vi "Configure AI.vi"(5 "Purpose (\"AI\")":string="AI", 7 "ADC #":T1=-1, 8 "error in (no error)":errorcluster, 11 "Session in":refnum<class "Session.lvclass">) -> (0 "error out":errorcluster, 3 "Session out":refnum<class "Session.lvclass">)   [LabVIEW 2024, in "CTI.lvlib" / "Session.lvclass"]
doc: "Configures a pin on the device to be used as an analog input. Unlike most other resource configuration VIs, the analog input is specified by its ADC number which can be found on the pinout for your device. Analog inputs are used to read a voltage value. When using these base AI features of the driver the raw integer reading will be returned which requires scaling to a proper voltage or engineering units and will depend on the wiring and configuration of the AI.\n\nThe Purpose input can be used to help with error reporting and provide a more specific intended use of the ADC that will be shown in future error messages resulting from I/O pin conflicts."
uses:
  Session.lvclass
  ADC Number.ctl
  Session.lvclass/Session.ctl
  2e1a53d0-5087-401c-a7a1-0aa9efa88061.vi
  Is Full Errors.vi
  Check Errors.vi
  CTI.lvlib
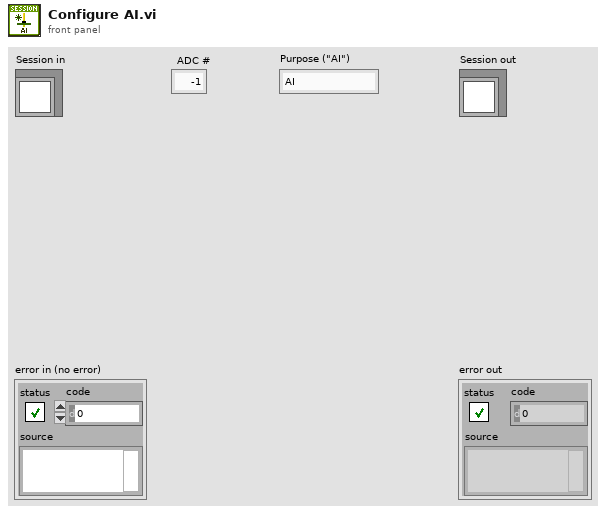
[diagram p1: front panel]
types:
  T1 = typedef "CTI.lvlib/ADC Number.ctl" = i8
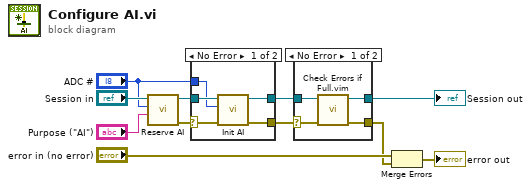
[diagram p0: block diagram]
diagram:
  n1 = call "Reserve AI.vi"("Purpose"="Purpose (\"AI\")", "ADC #"="ADC #", "Session in"="Session in") -> ("error out"=w4:errorcluster, "Session out"=w3:refnum<class "Session.lvclass">)  [unwired: 7 in]
  n2 = case shown="No Error" w4 {
    selector: w4 -> [w15 w17]
    tunnel: w3 -> [w16 w18]
    tunnel: [w14 w17] -> w11
    tunnel: [w13 w18] -> w10
    tunnel: "ADC #" -> [w12 _]
    frame No Error {
      n3 = call "Init AI.vi"("error in (no error)"=w15, "ADC #"=w12, "Session in"=w16) -> ("error out"=w14:errorcluster, "Session out"=w13:refnum<class "Session.lvclass">)  [unwired: 7 in]
    }
    frame Error {
    }
  }
  n4 = case shown="No Error" w11 {
    selector: w11 -> [w22 w24]
    tunnel: w10 -> [w20 w23]
    tunnel: [w21 w24] -> w7
    tunnel: [w19 w23] -> w9
    frame No Error {
      n5 = call "Check Errors if Full.vim"("error in (no error)"=w22, "Session in"=w20) -> ("error out"=w21:errorcluster, "Session out"=w19:refnum<class "Session.lvclass">)  [unwired: 8 in]
    }
    frame Error {
    }
  }
  "Session out" <- w9
  n6 = Merge Errors("error in (no error)", w7) -> (→"error out":errorcluster)
